vi "Prepare.vi"(8 "error in":errorcluster, 10 "Iterator Settings":T1={"Prepare timeout (ms)"=200, "Iterate timeout (ms)"=50, "Conclude timeout (ms)"=200, "Iterate period (ms)"=200, "Number of iterations"=5, "Time before stop (ms)"=5, "Active Stop Conditions"={"Number of Iterations"=FALSE, "Time Elapsed"=FALSE, "Iteration Result"=FALSE}, "Prepare Msg"=refnum, "Iterate Msg"=refnum, "Conclude Msg"=refnum, "Iterations End Report"=refnum}, 11 "Iterator Actor in":refnum<class "Iterator NR Actor.lvclass">) -> (0 "error out":errorcluster, 2 "Reply":bool, 3 "Iterator Actor out":refnum<class "Iterator NR Actor.lvclass">)   [LabVIEW 2023, in "Iterator Actor.lvlib" / "Iterator NR Actor.lvclass"]
doc: "Calls the Prepare method of the Client and receives its responce."
uses:
  Iterator NR Actor.lvclass
  Abstract Iterator Actor/Iterator Settings.ctl
  Iterator Actor/Iterator Actor Abstract Messages/Iterator Report Iterations End Msg/Iterator Report Iterations End Msg.lvclass
  <vilib>/ActorFramework/Message/Message.lvclass
  Abstract Iterator Actor/Active Stop Conditions.ctl
  Abstract Iterator Actor/Abstract Iterator Actor.lvclass/Abstract Iterator Actor.ctl
  <vilib>/ActorFramework/Actor/Actor.lvclass/Actor.ctl
  <vilib>/ActorFramework/Message Enqueuer/Message Enqueuer.lvclass/Message Enqueuer.ctl
  Abstract Iterator Actor/Iterator Errors.ctl
  Abstract Iterator Actor/Read Stop Iterate Notifier.vi
  <vilib>/ActorFramework/Message Priority Queue/Priority Enqueue.vi
  Iterator NR Actor.lvclass/Iterator NR Actor.ctl
  Abstract Iterator Actor/Abstract Iterator Actor.lvclass
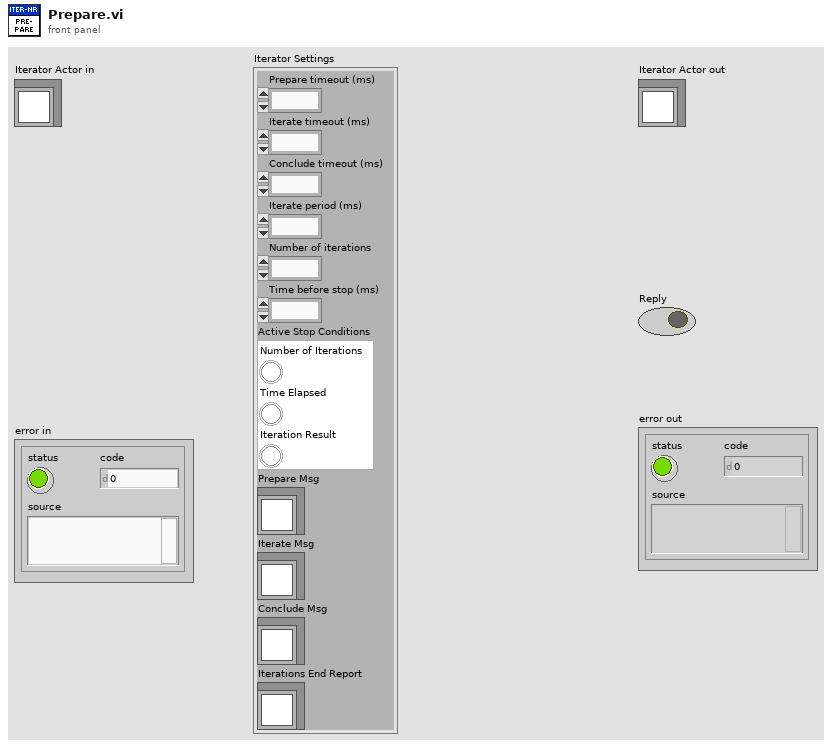
[diagram p1: front panel]
types:
  T1 = typedef "Iterator Actor.lvlib/Abstract Iterator Actor.lvclass/Iterator Settings.ctl" = cluster{"Prepare timeout (ms)":i32, "Iterate timeout (ms)":i32, "Conclude timeout (ms)":i32, "Iterate period (ms)":i32, "Number of iterations":i32, "Time before stop (ms)":i32, "Active Stop Conditions":T2, "Prepare Msg":refnum<class "Message.lvclass">, "Iterate Msg":refnum<class "Message.lvclass">, "Conclude Msg":refnum<class "Message.lvclass">, "Iterations End Report":refnum<class "Iterator Report Iterations End Msg.lvclass">}
  T2 = typedef "Iterator Actor.lvlib/Abstract Iterator Actor.lvclass/Active Stop Conditions.ctl" = cluster{"Number of Iterations":bool, "Time Elapsed":bool, "Iteration Result":bool}
  T3 = typedef "Iterator Actor.lvlib/Abstract Iterator Actor.lvclass/Iterator Errors.ctl" = enum16{"Input parameters are not valid", "Preparation call timed out", "Iteration call timed out", "Conclusion call timed out"}
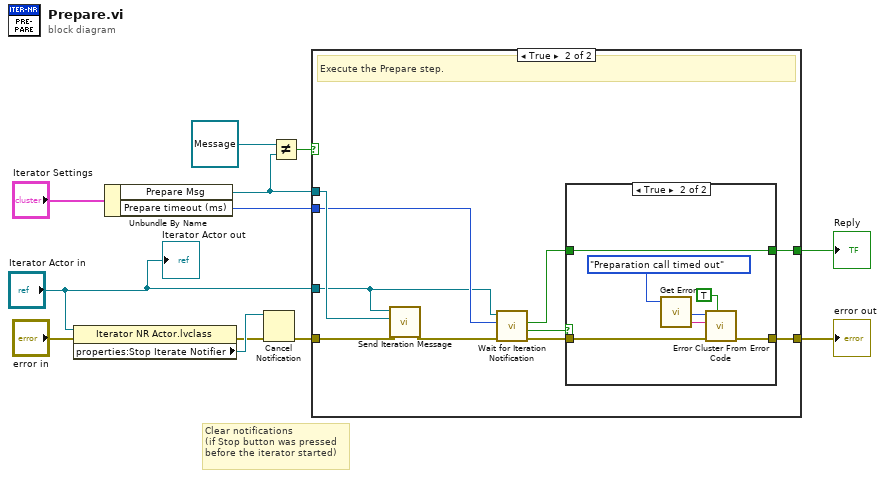
[diagram p0: block diagram]
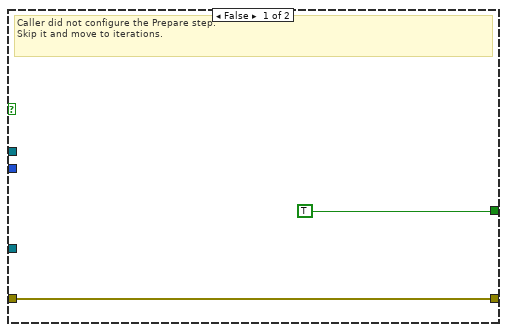
[diagram p2: hidden frame]
diagram:
  # "Clear notifications\n(if Stop button was pressed\nbefore the iterator started)"
  n1 = property class="Iterator NR Actor.lvclass"(reference="Iterator Actor in", error in="error in") -> (error out=w1:errorcluster, "properties:Stop Iterate Notifier"=w3:refnum<notifier>)  [unwired: 1 out]
  n2 = Unbundle By Name("Iterator Settings") -> ("Prepare Msg"=w5:refnum<class "Message.lvclass">, "Prepare timeout (ms)"=w12:i32)
  n3 = Cancel Notification(0:w3, 3:w1) -> (11:w9:errorcluster)  [unwired: 2 out]
  n4 = Not Equal?(x=refnum<class "Message.lvclass"> refnum ("Prepare Msg"), y=w5) -> (x != y?=w8:bool)
  n5 = case shown="True" w8 {
    tunnel: w12 -> [_ w18]
    tunnel: w5 -> [_ w24]
    tunnel: [TRUE w23] -> w7
    tunnel: [w14 w22] -> w10
    tunnel: w9 -> [w14 w21]
    tunnel: "Iterator Actor in" -> [_ w16]
    frame False {
      # "Caller did not configure the Prepare step.\nSkip it and move to iterations."
    }
    frame True {
      # "Execute the Prepare step."
      n6 = call "Send Iteration Message.vi"("error in (no error)"=w21, "Iteration Msg"=w24, "Iterator NR Actor in"=w16) -> ("error out"=w20:errorcluster)  [unwired: 8 in]
      n7 = call "Wait for Iteration Notification.vi"("error in (no error)"=w20, "timeout in ms (-1)"=w18, "Iterator NR Actor in"=w16) -> ("error out"=w19:errorcluster, "timed out?"=w17:bool, "Iterate?"=w15:bool)  [unwired: 5 in, 1 out]
      n8 = case shown="True" w17 {
        tunnel: w19 -> [w25 w30]
        tunnel: [w25 w29] -> w22
        tunnel: w15 -> [w26 w27]
        tunnel: [w26 w27] -> w23
        frame False {
        }
        frame True {
          n9 = call "Get Error.vi"("Error"=Iterator_Errors."Preparation call timed out") -> ("source"=w32:string, "code"=w31:i32)  [unwired: 2 in, 1 out]
          n10 = call <vilib>:"Error Cluster From Error Code.vi"("show call chain? (False)"=TRUE ("is warning? (False)"), "error in (no error)"=w30, "error message (\"\")"=w32, "error code (0)"=w31) -> ("error out"=w29:errorcluster)  [unwired: 5 in]
        }
      }
    }
  }
  "Reply" <- w7
  "error out" <- w10
  "Iterator Actor out" <- "Iterator Actor in"
